vi "Ograniczzenie zadanej predkości.vi"(11 "omega r[rad/s]":dbl) -> (3 "upper limit":dbl)   [LabVIEW 2012]
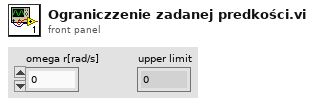
[diagram p1: front panel]
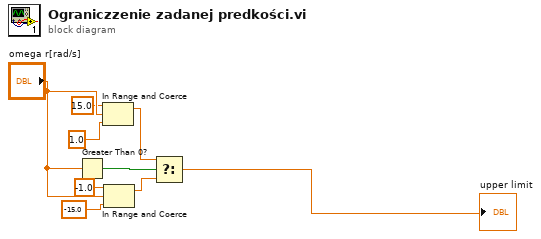
[diagram p0: block diagram]
diagram:
  n1 = Greater Than 0?(x="omega r[rad/s]") -> (x > 0?=w2:bool)
  n2 = In Range and Coerce(upper limit=15.0, x="omega r[rad/s]", lower limit=1.0) -> (coerced(x)=w9:dbl)  [unwired: 1 out]
  n3 = In Range and Coerce(upper limit=-1.0, x="omega r[rad/s]", lower limit=-15.0) -> (coerced(x)=w4:dbl)  [unwired: 1 out]
  n4 = Select(t=w9, s=w2, f=w4) -> (s? t:f=→"upper limit":dbl)
